vi "Async VI Control_Run Process.vi"(6 "Parent VI":refnum<vi>, 8 "error in (no error)":errorcluster, 10 "Initial Parameters":cluster{"Initial Parameters":T1[]}[](array[cluster]), 11 "VI Ref In":refnum<vi>[](array[refnum])) -> (0 "error out":errorcluster, 3 "VI Ref In":refnum<vi>[](array[refnum]))   [LabVIEW 2013, in "CANOpen Addon Custom Device.lvlib"]
uses:
  CANOpen Addon Custom Device.lvlib
  _Controls/Async VI Control_Parameters Cluster.ctl
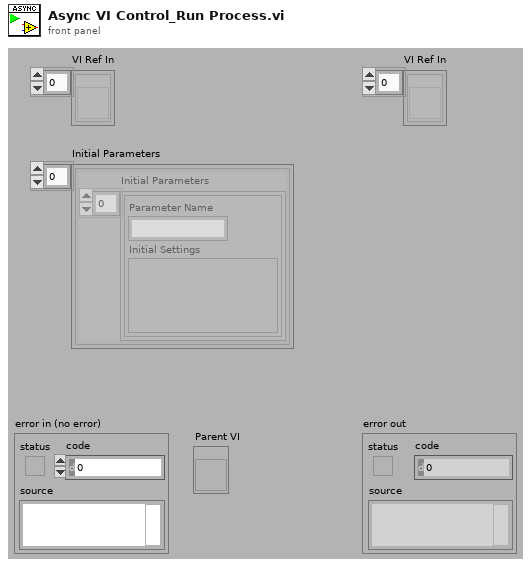
[diagram p1: front panel]
types:
  T1 = typedef "CANOpen Addon Custom Device.lvlib/Async VI Control_Parameters Cluster.ctl" = cluster{"Parameter Name":string, "Initial Settings":variant}
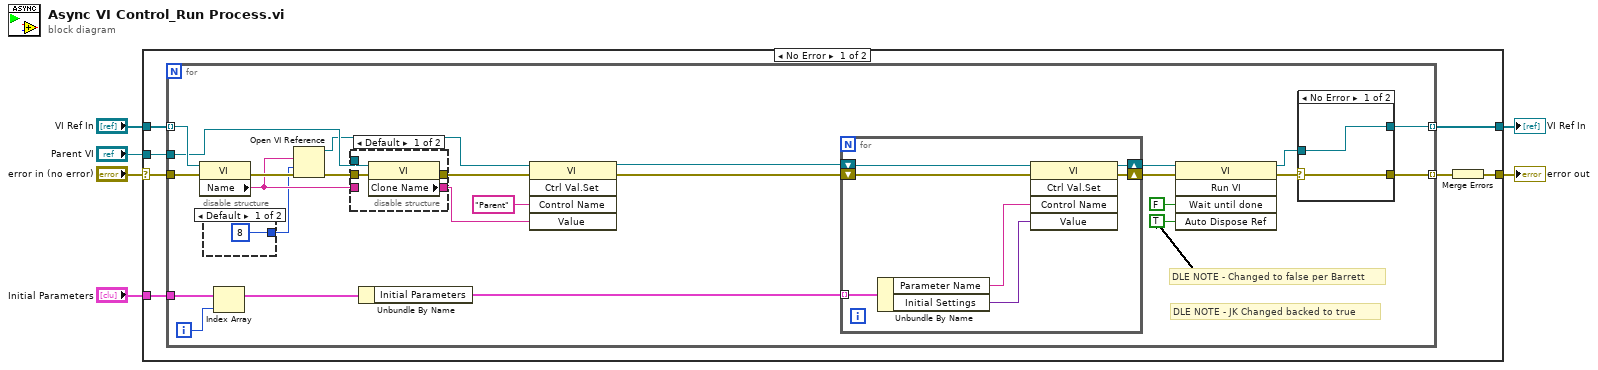
[diagram p0: block diagram]
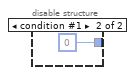
[diagram p2: hidden frame]
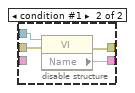
[diagram p3: hidden frame]
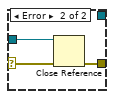
[diagram p4: hidden frame]
diagram:
  n1 = case shown="No Error" "error in (no error)" {
    selector: "error in (no error)" -> [w10 w62]
    tunnel: [w7 w62] -> w6
    tunnel: "VI Ref In" -> [w12 w61]
    tunnel: [w11 w61] -> w4
    tunnel: "Initial Parameters" -> [w8 _]
    tunnel: "Parent VI" -> [w9 _]
    frame No Error {
      n2 = for {
        tunnel: [w38] -> w13 mode=indexing
        tunnel: w12 -> [w37] mode=indexing
        tunnel: [w36] -> w11 mode=indexing
        tunnel: w10 -> [w23]
        tunnel: w9 -> [w22]
        tunnel: w8 -> [w27]
        i -> [w24]
        # "DLE NOTE - JK Changed backed to true"
        # "DLE NOTE - Changed to false per Barrett"
        n3 = property class="VI"(reference=w37, error in=w23) -> (error out=w29:errorcluster, "Name"=w18:string)  [unwired: 1 out]
        n4 = disable-structure shown="Default" {
          disable-tunnel: [8 ("options") 0 ("options")] -> w16
          frame condition #0 (active) {
          }
          frame condition #1 {
          }
        }
        n5 = Index Array(array=w27, index=w24) -> (element=w25:cluster{"Initial Parameters":T1[]})
        n6 = Open VI Reference(vi path=w18, options=w16, error in (no error)=w29) -> (vi reference=w17:refnum<vi>, error out=w21:errorcluster)  [unwired: 3 out]
        n7 = disable-structure shown="Default" {
          disable-tunnel: w22 -> [w44 w48]
          disable-tunnel: w21 -> [w43 w47]
          disable-tunnel: [w42 w46] -> w20
          disable-tunnel: [w41 w45] -> w19
          disable-tunnel: w18 -> [_ _]
          frame condition #0 (active) {
            n8 = property class="VI"(reference=w44, error in=w43) -> (error out=w41:errorcluster, "Clone Name"=w42:string)  [unwired: 1 out]
          }
          frame condition #1 {
            n9 = property class="VI"(reference=w48, error in=w47) -> (error out=w45:errorcluster, "Name"=w46:string)  [unwired: 1 out]
          }
        }
        n10 = Unbundle By Name(w25) -> ("Initial Parameters"=w26:T1[])
        n11 = invoke class="VI" method="Ctrl Val.Set"(reference=w17, error in=w19, "Control Name"="Parent", "Value"=w20) -> (reference out=w15:refnum<vi>, error out=w14:errorcluster)  [unwired: 1 in, 3 out]
        n12 = for {
          tunnel: w26 -> [w51] mode=indexing
          shift-right: [w54] -> w30
          shift-left: w15 -> [w52]
          shift-right: [w55] -> w31
          shift-left: w14 -> [w53]
          n13 = Unbundle By Name(w51) -> ("Parameter Name"=w50:string, "Initial Settings"=w49:variant)
          n14 = invoke class="VI" method="Ctrl Val.Set"(reference=w52, error in=w53, "Control Name"=w50, "Value"=w49) -> (reference out=w54:refnum<vi>, error out=w55:errorcluster)  [unwired: 1 in, 3 out]
        }
        n15 = invoke class="VI" method="Run VI"(reference=w30, error in=w31, "Wait until done"=FALSE ("Wait Until Done"), "Auto Dispose Ref"=TRUE ("Auto Dispose Reference")) -> (reference out=w32:refnum<vi>, error out=w33:errorcluster)  [unwired: 1 in, 3 out]
        n16 = case shown="No Error" w33 {
          selector: w33 -> [w57 w60]
          tunnel: w32 -> [w56 w59]
          tunnel: [w57 w58] -> w38
          tunnel: [w56 _] -> w36
          frame No Error {
          }
          frame Error {
            n17 = Close Reference(reference=w59, error in (no error)=w60) -> (error out=w58:errorcluster)
          }
        }
      }
      n18 = Merge Errors(w13) -> (w7:errorcluster)
    }
    frame Error {
    }
  }
  "error out" <- w6
  "VI Ref In" <- w4
